vi "DIO In Get Refnum (Water Tank).vi"(8 "error in (no error)":errorcluster, 10 "refnum name":string="My DigitalInput RefNum") -> (0 "error out":errorcluster, 3 "DigitalInputDevRef":cluster{string, i32})   [LabVIEW 2013]
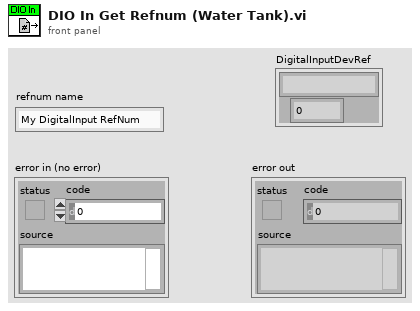
[diagram p1: front panel]
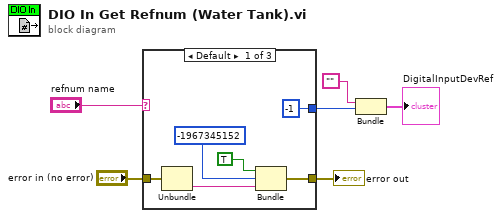
[diagram p0: block diagram]
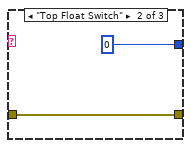
[diagram p2: hidden frame]
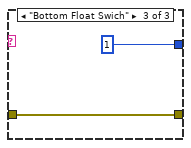
[diagram p3: hidden frame]
diagram:
  n1 = case shown="Default" "refnum name" {
    tunnel: "error in (no error)" -> [w12 w14 w16]
    tunnel: [w7 w14 w16] -> w4
    tunnel: [-1 0 1] -> w2
    frame Default {
      n2 = Unbundle(w12) -> ("source"=w8:string)  [unwired: 2 out]
      n3 = Bundle(TRUE, -1967345152, "source"=w8) -> (w7:cluster{bool, i32, "source":string})  [unwired: 1 in]
    }
    frame "Top Float Switch" {
    }
    frame "Bottom Float Swich" {
    }
  }
  "error out" <- w4
  n4 = Bundle("", w2) -> (→"DigitalInputDevRef":cluster{string, i32})  [unwired: 1 in]
